vi "Overlay Image with Sector ROI.vi"(7 "FPGA Display Image In":T1=refnum, 8 "error in":errorcluster, 11 "FPGA Image":T1=refnum) -> (0 "error out":errorcluster, 3 "FPGA Display Image Out":T1)   [LabVIEW 2013]
uses:
  <vilib>/vision/Image Controls.llb/IMAQ Image.ctl
  Image Processing/Mask ROI FG Enum.ctl
  Globals/Average Sector Data.vi
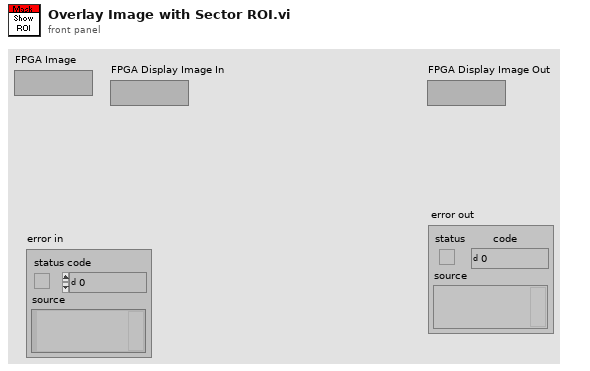
[diagram p1: front panel]
types:
  T1 = typedef "IMAQ Image.ctl" = refnum<image>
  T2 = typedef "Mask ROI FG Enum.ctl" = enum16{"Read", "Write", "Enable Background", "Disable Background"}
  T3 = typedef "Mask ROI Cluster.ctl" = cluster{"left annulus":T4, "right annulus":T4, "Threshold Range":cluster{"Lower value":dbl, "Upper value":dbl}, "[Avg BG]":u8[], "Number of Sectors":u8, "Left ROI":T5, "Right ROI":T5, "Left Start Angle Duty Cycle":fxp<+,8,0>, "Left End Angle Duty Cycle":fxp<+,8,0>, "Right End Angle Duty Cycle":fxp<+,8,0>, "Right Start Angle Duty Cycle":fxp<+,8,0>, "[Sector ROIs]":T5[], "Consecutive Sector Threshold":u8}
  T4 = typedef "IMAQ Circle" = cluster{"Center X":i32, "Center Y":i32, "Inner Radius":i32, "Outer Radius":i32, "Start Angle":dbl, "End Angle":dbl}
  T5 = typedef "ROI Descriptor" = cluster{"Global Rectangle":i32[], "Contours":cluster{"ID":enum32{"External", "Internal"}, "Type":u32, "Coordinates":i32[]}[]}
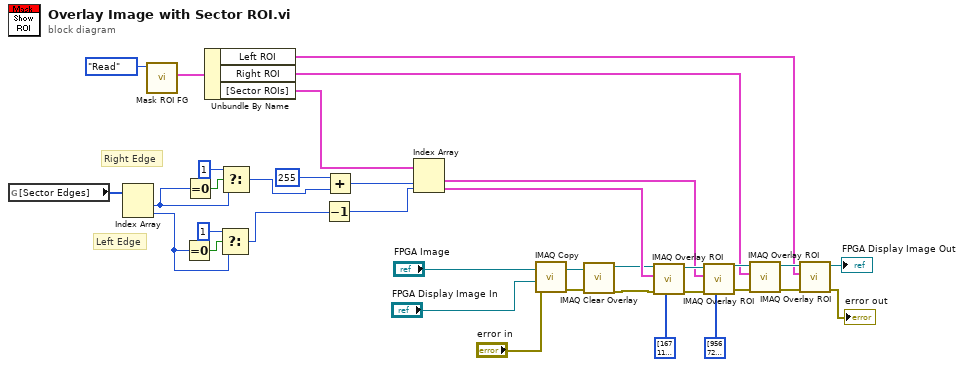
[diagram p0: block diagram]
diagram:
  # "Left Edge"
  # "Right Edge"
  n1 = global read "Average Sector Data.vi" "[Sector Edges]"() -> (w16:u16[])
  n2 = Index Array(array=w16) -> (element #1=w4:u16, element #2=w1:u16)  [unwired: 2 in]
  n3 = call "Mask ROI FG.vi"("Operation"=Mask_ROI_FG_Enum."Read") -> ("Mask ROI Out"=w21:T3)  [unwired: 9 in, 1 out]
  n4 = Equal To 0?(x=w1) -> (x = 0?=w5:bool)
  n5 = Equal To 0?(x=w4) -> (x = 0?=w7:bool)
  n6 = Unbundle By Name(w21) -> ("Left ROI"=w20:T5, "Right ROI"=w19:T5, "[Sector ROIs]"=w18:T5[])
  n7 = Select(t=u16 1, s=w5, f=w1) -> (s? t:f=w2:u16)
  n8 = Select(t=u16 1, s=w7, f=w4) -> (s? t:f=w3:u16)
  n9 = Decrement(x=w2) -> (x-1=w30:u16)
  n10 = Add(x=u16 255, y=w3) -> (x+y=w31:u16)
  n11 = Index Array(array=w18, index #1=w31, index #2=w30) -> (element #1=w22:T5, element #2=w23:T5)
  n12 = call "IMAQ Copy"("error in (no error)"="error in", "Image Dst"="FPGA Display Image In", "Image Src"="FPGA Image") -> ("error out"=w14:errorcluster, "Image Dst Out"=w13:T1)  [unwired: 3 in]
  n13 = call "IMAQ Clear Overlay"("error in (no error)"=w14, "Image"=w13) -> ("error out"=w11:errorcluster, "Image Out"=w12:T1)  [unwired: 8 in]
  n14 = call "IMAQ Overlay ROI"("Colors (Green)"=u32[] [16711935], "error in (no error)"=w11, "ROI Descriptor"=w23, "Image"=w12) -> ("error out"=w36:errorcluster, "Image Out"=w35:T1)  [unwired: 6 in]
  n15 = call "IMAQ Overlay ROI"("Colors (Green)"=u32[] [9567230], "error in (no error)"=w36, "ROI Descriptor"=w22, "Image"=w35) -> ("error out"=w24:errorcluster, "Image Out"=w28:T1)  [unwired: 6 in]
  n16 = call "IMAQ Overlay ROI"("error in (no error)"=w24, "ROI Descriptor"=w19, "Image"=w28) -> ("error out"=w29:errorcluster, "Image Out"=w27:T1)  [unwired: 7 in]
  n17 = call "IMAQ Overlay ROI"("error in (no error)"=w29, "ROI Descriptor"=w20, "Image"=w27) -> ("error out"=→"error out":errorcluster, "Image Out"=→"FPGA Display Image Out":T1)  [unwired: 7 in]
